vi "RemoveShapeByRef Response.vi"(8 "error in (no error)":errorcluster, 10 "Shape to Remove":refnum<data-value>, 11 "Image Editor Handler in":refnum<class "Image Editor Handler.lvclass">) -> (0 "error out":errorcluster, 3 "Image Editor Handler out":refnum<class "Image Editor Handler.lvclass">)   [LabVIEW 2017, in "LV Image Editor Framework.lvlib" / "Image Editor Handler.lvclass"]
uses:
  <vilib>/LIEF/Image Editor Handler/Image Editor Handler.lvclass
  <vilib>/LIEF/Forms/Shape/Shape.lvclass
  <vilib>/LIEF/Image Editor Handler/Image Editor Handler.lvclass/Image Editor Handler.ctl
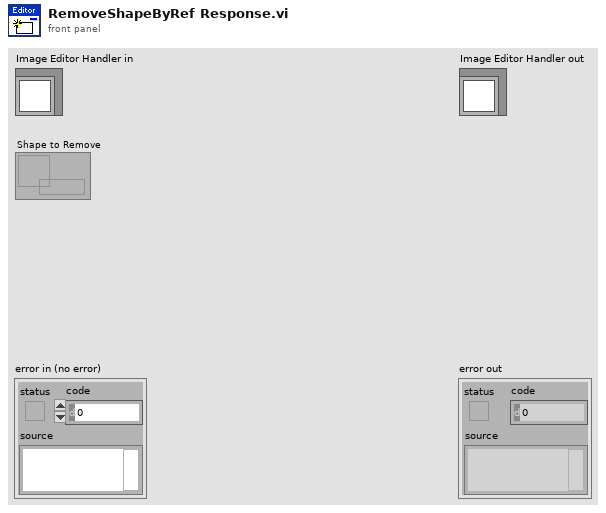
[diagram p1: front panel]
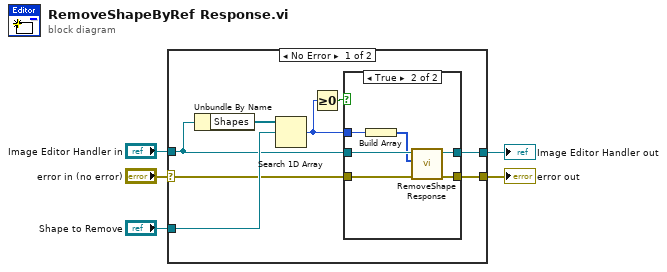
[diagram p0: block diagram]
diagram:
  n1 = case shown="No Error" "error in (no error)" {
    selector: "error in (no error)" -> [w8 w23]
    tunnel: [w7 w23] -> w4
    tunnel: [w6 w22] -> w2
    tunnel: "Image Editor Handler in" -> [w9 w22]
    tunnel: "Shape to Remove" -> [w13 _]
    frame No Error {
      n2 = Unbundle By Name(w9) -> ("Shapes"=w12:refnum<data-value>[])
      n3 = Search 1D Array(1D array=w12, element=w13) -> (index of element=w11:i32)  [unwired: 1 in]
      n4 = Greater Or Equal To 0?(x=w11) -> (x >= 0?=w10:bool)
      n5 = case shown="True" w10 {
        tunnel: w11 -> [_ w21]
        tunnel: w9 -> [w14 w20]
        tunnel: w8 -> [w15 w18]
        tunnel: [w15 w17] -> w7
        tunnel: [w14 w16] -> w6
        frame False {
        }
        frame True {
          n6 = Build Array(w21) -> (w19:i32[])
          n7 = call-dynamic "RemoveShape Response.vi"("error in (no error)"=w18, "Indexes"=w19, "Image Editor Handler in"=w20) -> ("error out"=w17:errorcluster, "Image Editor Handler out"=w16:refnum<class "Image Editor Handler.lvclass">)  [unwired: 7 in]
        }
      }
    }
    frame Error {
    }
  }
  "error out" <- w4
  "Image Editor Handler out" <- w2
